vi "Close.vi"(8 "error in (no error)":errorcluster caption="entrée d'erreur (pas d'erreur)", 11 "Class Balance_Adam_GBK en entrée":refnum<class "Class Balance_Adam_GBK.lvclass">) -> (0 "error out":errorcluster caption="sortie d'erreur", 3 "Class Balance_Adam_GBK en sortie":refnum<class "Class Balance_Adam_GBK.lvclass">)   [LabVIEW 2020, in "Library Instrument & Equipement.lvlib" / "Library Balance.lvlib" / "Class Balance_Adam_GBK.lvclass"]
uses:
  Class Balance_Adam_GBK.lvclass
  C:/Users/ngarcin/OneDrive - Altyor/Standard TB/Class/Balance/Balance (Default)/Class Balance (Default).lvclass
  Class Balance_Adam_GBK.lvclass/Class Balance_Adam_GBK.ctl
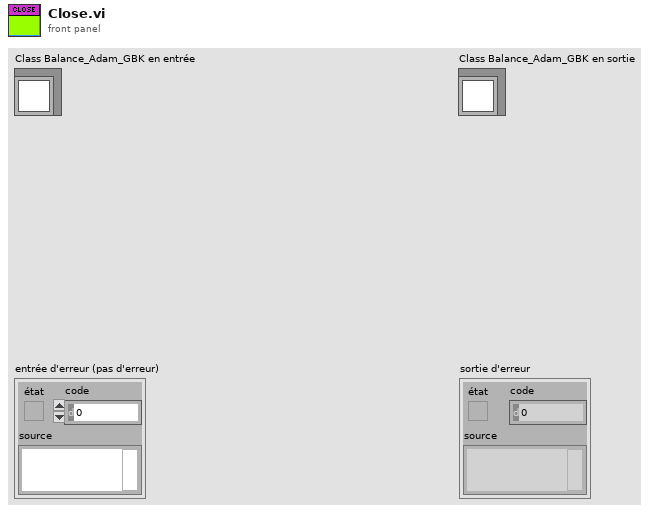
[diagram p1: front panel]
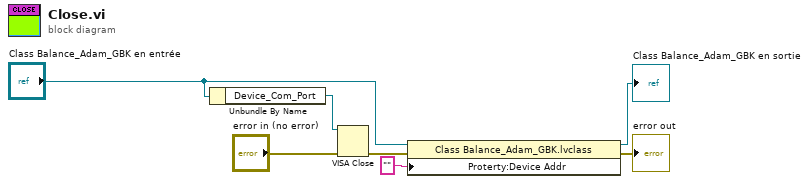
[diagram p0: block diagram]
diagram:
  n1 = Unbundle By Name("Class Balance_Adam_GBK en entrée") -> ("Device_Com_Port"=w3:refnum<visa-resource-name>)
  n2 = VISA Close(VISA resource name=w3, error in (no error)="error in (no error)") -> (error out=w7:errorcluster)
  n3 = property class="Class Balance_Adam_GBK.lvclass"(reference="Class Balance_Adam_GBK en entrée", error in=w7, "Proterty:Device Addr"="" ("Address_Device")) -> (reference out=→"Class Balance_Adam_GBK en sortie":refnum<class "Class Balance_Adam_GBK.lvclass">, error out=→"error out":errorcluster)
